vi "Convert Times to Interval and Span.vi"(8 "Time Bucket":T1=enum."1 second", 9 "End":timestamp, 10 "Start":timestamp) -> (0 "Time Bucket out":T1, 1 "Span":dbl, 2 "time interval":T2)   [LabVIEW 2019, in "Database Viewer.lvclass"]
uses:
  Database Viewer.lvclass
  typedefs/Time Bucket--enum.ctl
panel:
  out "step":dbl
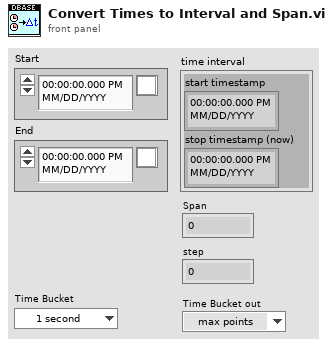
[diagram p1: front panel]
types:
  T1 = typedef "Database Viewer.lvclass/Time Bucket--enum.ctl" = enum16{"max points", "automatic", "1 second", "10 seconds", "1 minute", "10 minutes", "1 hour", "10 hours", "1 day", "10 days"}
  T2 = cluster{"start timestamp":timestamp, "stop timestamp (now)":timestamp}
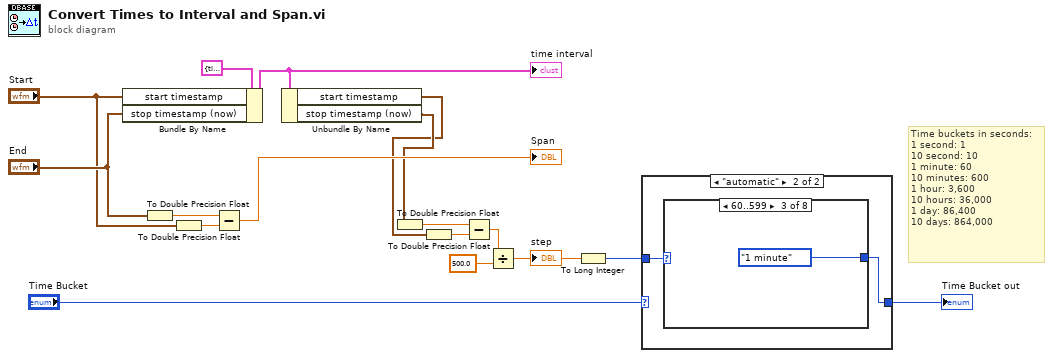
[diagram p0: block diagram]
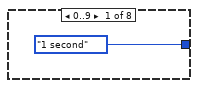
[diagram p3: hidden frame]
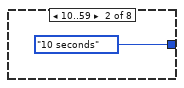
[diagram p4: hidden frame]
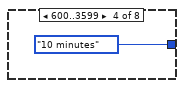
[diagram p5: hidden frame]
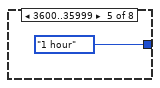
[diagram p6: hidden frame]
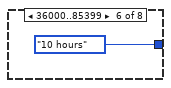
[diagram p7: hidden frame]
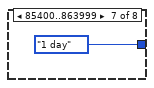
[diagram p8: hidden frame]
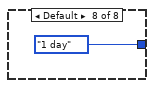
[diagram p9: hidden frame]
diagram:
  # "Time buckets in seconds:\n1 second: 1\n10 second: 10\n1 minute: 60\n10 minutes: 600\n1 hour: 3,600\n10 hours: 36,000\n1 day: 86,400\n10 days: 864,000"
  n1 = Bundle By Name(cluster=T2 {"start timestamp"=timestamp(0 s since 1904-01-01), "stop timestamp (now)"=timestamp(0 s since 1904-01-01)} ("time interval"), "start timestamp"="Start", "stop timestamp (now)"="End") -> (w6:T2)
  "time interval" <- w6
  n2 = To Double Precision Float(number="End") -> (double precision float=w14:dbl)
  n3 = To Double Precision Float(number="Start") -> (double precision float=w13:dbl)
  n4 = Subtract(x=w14, y=w13) -> (x-y=→"Span":dbl)
  n5 = Unbundle By Name(w6) -> ("start timestamp"=w2:timestamp, "stop timestamp (now)"=w3:timestamp)
  n6 = To Double Precision Float(number=w3) -> (double precision float=w4:dbl)
  n7 = To Double Precision Float(number=w2) -> (double precision float=w5:dbl)
  n8 = Subtract(x=w4, y=w5) -> (x-y=w1:dbl)
  n9 = Divide(x=w1, y=500.0) -> (x/y=w10:dbl)
  "step" <- w10
  n10 = To Long Integer(number=w10) -> (32bit integer=w9:i32)
  n11 = case shown="\"automatic\"" "Time Bucket" {
    selector: "Time Bucket" -> [w18 _]
    tunnel: w9 -> [_ w20]
    tunnel: [w18 w19] -> w7
    frame Default {
    }
    frame "automatic" {
      n12 = case shown="60..599" w20 {
        tunnel: [Time_Bucket--enum."1 second" ("Time Bucket") Time_Bucket--enum."10 seconds" ("Time Bucket") Time_Bucket--enum."1 minute" ("Time Bucket") Time_Bucket--enum."10 minutes" ("Time Bucket") Time_Bucket--enum."1 hour" ("Time Bucket") Time_Bucket--enum."10 hours" ("Time Bucket") Time_Bucket--enum."1 day" ("Time Bucket") Time_Bucket--enum."1 day" ("Time Bucket")] -> w19
        frame 0..9 {
        }
        frame 10..59 {
        }
        frame 60..599 {
        }
        frame 600..3599 {
        }
        frame 3600..35999 {
        }
        frame 36000..85399 {
        }
        frame 85400..863999 {
        }
        frame Default {
        }
      }
    }
  }
  "Time Bucket out" <- w7
